vi "Transmit - UDP (SAP).vi"() -> ()   [LabVIEW 2020]
uses:
  <instrlib>/AIM GmbH/_AIM 664/_controls/comm_config_vl_tx.ctl
  <instrlib>/AIM GmbH/_AIM 664/_controls/sap_config_tx.ctl
  <instrlib>/AIM GmbH/_AIM 664/helpers/EthFrameManagement/controls/mac_src_info_afdx.ctl
  <instrlib>/AIM GmbH/_AIM 664/_polimorphicInstances/session/CreateSession(Tx-UDP Port-Oriented).vi
  <instrlib>/AIM GmbH/_AIM 664/bsp/AFDX_Transmit/Create Tx VL.vi
  <instrlib>/AIM GmbH/_AIM 664/_polimorphicInstances/udpPort/CreateUdpPort(TX-SAP).vi
  <instrlib>/AIM GmbH/_AIM 664/_polimorphicInstances/control/Start (Tx).vi
  <instrlib>/AIM GmbH/_AIM 664/_polimorphicInstances/control/Stop (Tx).vi
  <instrlib>/AIM GmbH/_AIM 664/_polimorphicInstances/session/CleanupSession (Port).vi
  <instrlib>/AIM GmbH/_AIM 664/AIM664LV.lvlib
  <instrlib>/AIM GmbH/_AIM 664/helpers/EthFrameManagement/EthFrameManagement.lvlib
panel:
  in  "source info":T1
  in  "Period mS":u32=200
  in  "SapPort Config":T2={"partitionID"=0, "SubVlId"=0, "UdpSrcPort"=1, "UdpNumBufMessages"=0, "UdpMaxMessageSize"=1000}
  in  "VL Config":T3={"VlId"=30, "NumOfSubVl"=1, "rate mS (128)"=128.0, "domainID"=1, "sideID"=1, "locationID"=1, "interfaceID"=1, "NetSelect"=3, "Skew"=0, "MaxFrameLength"=1000, "FrameBufferSize"=0} {"NetSelect" items=["FDX_TX_FRAME_DLY_A"=0, "FDX_TX_FRAME_DLY_B"=1, "FDX_TX_FRAME_BOTH "=3, "FDX_TX_FRAME_ONLY_A"=4, "FDX_TX_FRAME_ONLY_B "=5]; "interfaceID" format="%.0b"}
  out "BytesWritten":u32
  out "Curent Irig Time":T4
  out "CurrentIndex":u32
  out "MsgCount":u32
  out "IndexCycleCount":u32
  in  "VLid Dest":u32=30
  in  "UdpDst":u32=12345
  in  "Data":u8[](array[numeric])=[10, 10, 10, 10, 10, 10, 10, 10, 10, 10, 10, 10, 10, 10, 10, 10, 10, 10, 10, 10, 10, 10, 10, 10, 10, 10, 10, 10, 10, 10, 10, 10, 10, 10, 10, 10, 10, 10, 10, 10, 10, 10, 10, 10, 10, 10, 10, 10, 10, 10, 10, 10, 10, 10, 10, 10, 10, 10, 10, 10, 10, 10, 10, 10, 10, 10, 10, 10, 10, 10, 10, 10, 10, 10, 10, 10, 10, 10, 10, 10, 10, 10, 10, 10, 10, 10, 10, 10, 10, 10, 10, 10, 10, 10, 10, 10, 10, 10, 10, 15] format="%.0x"
  out "PortInitOut":T5 {"PortConfig" items=["FDX_SINGLE", "FDX_REDUNDANT"]}
  in  "port":u32
  in  "board":u32=1
  out "error out":errorcluster
  in  "stop":bool
  out "current time":timestamp
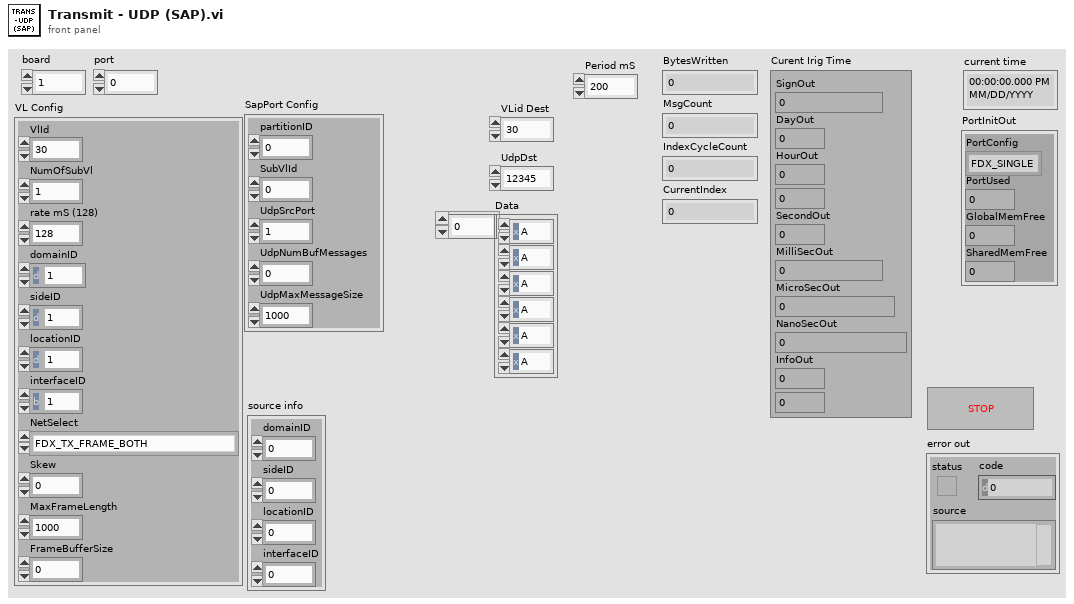
[diagram p1: front panel]
types:
  T1 = typedef "EthFrameManagement.lvlib/mac_src_info_afdx.ctl" = cluster{"domainID":u8, "sideID":u8, "locationID":u8, "interfaceID":u8}
  T2 = typedef "AIM664LV.lvlib/sap_config_tx.ctl" = cluster{"partitionID":u8, "SubVlId":u8, "UdpSrcPort":u16, "UdpNumBufMessages":u32, "UdpMaxMessageSize":u32}
  T3 = typedef "AIM664LV.lvlib/comm_config_vl_tx.ctl" = cluster{"VlId":u16, "NumOfSubVl":u16, "rate mS (128)":dbl, "domainID":u8, "sideID":u8, "locationID":u8, "interfaceID":u8, "NetSelect":u32, "Skew":u32, "MaxFrameLength":u32, "FrameBufferSize":u32}
  T4 = cluster{"SignOut":i32, "DayOut":u32, "HourOut":u32, "MinOut":u32, "SecondOut":u32, "MilliSecOut":u32, "MicroSecOut":u32, "NanoSecOut":u32, "InfoOut":u32, "Mode":u32}
  T5 = cluster{"PortConfig":u32, "PortUsed":u32, "GlobalMemFree":u32, "SharedMemFree":u32}
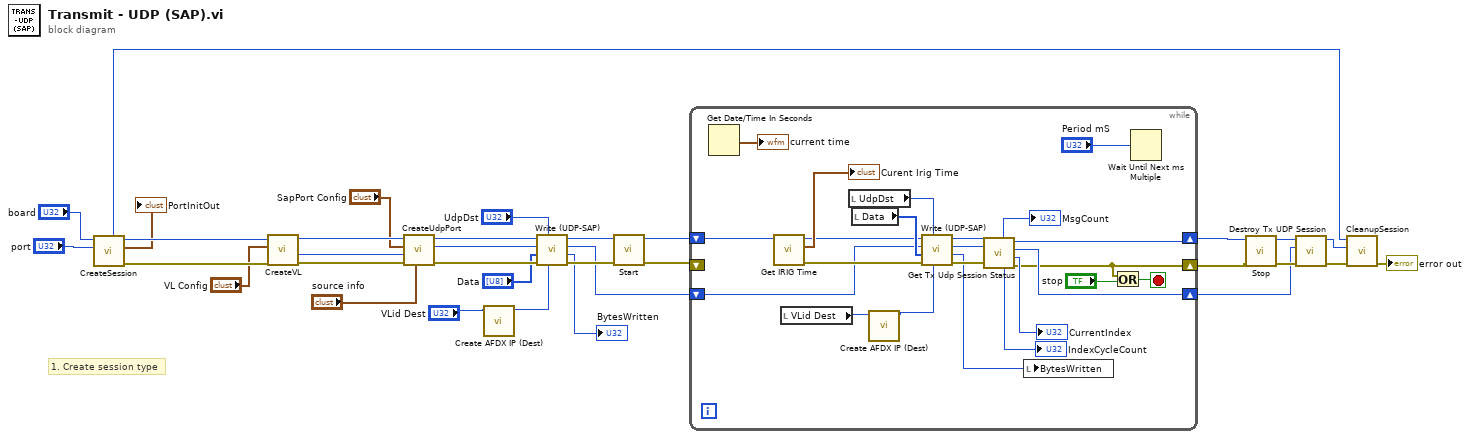
[diagram p0: block diagram]
diagram:
  # "1. Create session type"
  n1 = call-poly <instrlib>:"CreateSession.vi"("port"="port", "board"="board") -> ("error out"=w32:errorcluster, "PortInitOut"=→"PortInitOut":T5, "port handle out"=w33:u32, "InstrumentHandle_board out"=w4:u32)  [unwired: 5 in, 1 out]
  n2 = call-poly <instrlib>:"CreateVL.vi"("error in (no error)"=w32, "VL Config"="VL Config", "InstrumentHandle in"=w33) -> ("error out"=w30:errorcluster, "VlId"=w19:u16, "InstrumentHandle out"=w31:u32)  [unwired: 6 in]
  n3 = call-poly <instrlib>:"CreateUdpPort.vi"("source info"="source info", "error in (no error)"=w30, "VlId"=w19, "SapPort Config"="SapPort Config", "port handle in"=w31) -> ("error out"=w22:errorcluster, "sapPort handle out"=w9:u32, "port handle out"=w14:u32)  [unwired: 3 in, 1 out]
  n4 = call <instrlib>:"Create AFDX IP (Dest).vi"("VL"="VLid Dest") -> ("ip net"=w15:u32)  [unwired: 9 in, 1 out]
  n5 = call <instrlib>:"Write (UDP-SAP).vi"("IpDst"=w15, "UdpDst"="UdpDst", "error in (no error)"=w22, "Data"="Data", "UdpHandle in"=w9, "InstrumentHandle_port in"=w14) -> ("error out"=w23:errorcluster, "BytesWritten"=→"BytesWritten":u32, "UdpHandle out"=w11:u32, "InstrumentHandle_port out"=w12:u32)  [unwired: 2 in]
  n6 = call-poly <instrlib>:"Start.vi"("error in (no error)"=w23, "InstrumentHandle_port in"=w12) -> ("error out"=w2:errorcluster, "InstrumentHandle_port out"=w29:u32)  [unwired: 8 in]
  n7 = while {
    shift-right: [w40] -> w28
    shift-left: w29 -> [w53]
    shift-right: [w39] -> w7
    shift-left: w11 -> [w43]
    shift-right: [w34] -> w3
    shift-left: w2 -> [_]
    stop <- w36 stop-if-true
    n8 = Get Date/Time In Seconds() -> (seconds since 1Jan1904=→"current time":timestamp)
    n9 = call <instrlib>:"Get IRIG Time.vi"("InstrumentHandle_board in"=w53) -> ("error out"=w52:errorcluster, "Curent Irig Time"=→"Curent Irig Time":T4, "InstrumentHandle_board out"=w38:u32)  [unwired: 8 in]
    n10 = local read "VLid Dest"() -> (w45:u32)
    n11 = local read "UdpDst"() -> (w48:u32)
    n12 = local read "Data"() -> (w47:u8[])
    n13 = call <instrlib>:"Create AFDX IP (Dest).vi"("VL"=w45) -> ("ip net"=w46:u32)  [unwired: 9 in, 1 out]
    n14 = call <instrlib>:"Write (UDP-SAP).vi"("IpDst"=w46, "UdpDst"=w48, "error in (no error)"=w52, "Data"=w47, "UdpHandle in"=w43, "InstrumentHandle_port in"=w38) -> ("error out"=w50:errorcluster, "BytesWritten"=w44:u32, "UdpHandle out"=w42:u32, "InstrumentHandle_port out"=w49:u32)  [unwired: 2 in]
    n15 = call <instrlib>:"Get Tx Udp Session Status.vi"("error in (no error)"=w50, "UdpHandle in"=w42, "InstrumentHandle_port in"=w49) -> ("error out"=w34:errorcluster, "CurrentIndex"=→"CurrentIndex":u32, "UdpHandle out"=w39:u32, "InstrumentHandle_port out"=w40:u32, "IndexCycleCount"=→"IndexCycleCount":u32, "MsgCount"=→"MsgCount":u32)  [unwired: 3 in]
    n16 = local write "BytesWritten"(w44) -> ()
    n17 = Or(x=w34, y="stop") -> (x .or. y?=w36:bool)
    n18 = Wait Until Next ms Multiple(millisecond multiple="Period mS") -> ()  [unwired: 1 out]
  }
  n19 = call-poly <instrlib>:"Stop.vi"("error in (no error)"=w3, "InstrumentHandle_port in"=w28) -> ("error out"=w21:errorcluster, "InstrumentHandle_port out"=w6:u32)  [unwired: 8 in]
  n20 = call <instrlib>:"Destroy Tx UDP Session.vi"("error in (no error)"=w21, "UdpHandle in"=w7, "InstrumentHandle_port in"=w6) -> ("error out"=w20:errorcluster, "InstrumentHandle_port out"=w5:u32)  [unwired: 7 in]
  n21 = call-poly <instrlib>:"CleanupSession.vi"("error in (no error)"=w20, "InstrumentHandle_port in"=w5, "InstrumentHandle_board in"=w4) -> ("error out"=→"error out":errorcluster)  [unwired: 8 in]
